vi "Transmit Module Command.vi"(8 "error in":errorcluster, 11 "SL_SC in":refnum<class "SL_SC.lvclass">) -> (0 "error out":errorcluster, 3 "SL_SC out":refnum<class "SL_SC.lvclass">)   [LabVIEW 2019, in "SL_SC.lvlib" / "SL_SC.lvclass"]
uses:
  Library/SL_SC.lvclass
  C:/Users/Public/Documents/Development/builds/Instruments/DIG_IO.lvlibp/Library/DIG_IO.lvclass
  Library/SL_SC.lvclass/SL_SC.ctl
  builds/Instruments/DIG_IO.lvlibp/Accessors/Read Digital.vi
  <vilib>/SLSC/Set Device Property (U32).vi
  <vilib>/SLSC/Commit Properties for Devices.vi
  <vilib>/SLSC/SLSC.lvlib
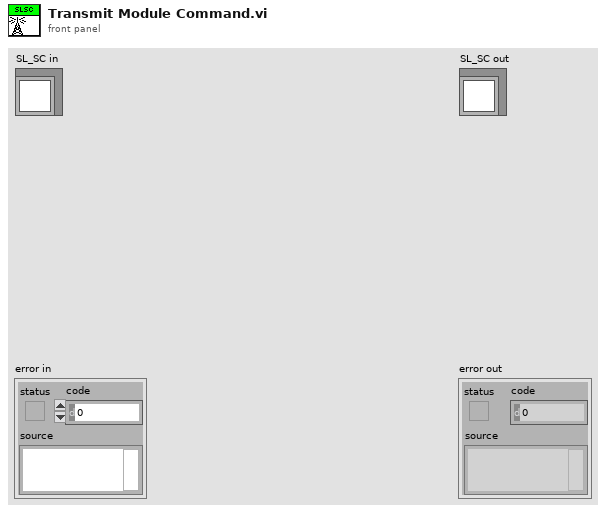
[diagram p1: front panel]
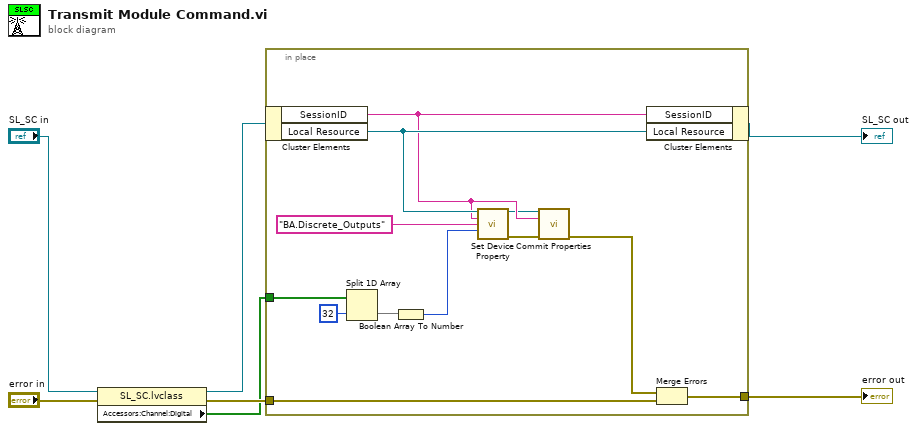
[diagram p0: block diagram]
diagram:
  n1 = property class="SL_SC.lvclass"(reference="SL_SC in", error in="error in") -> (reference out=w2:refnum<class "SL_SC.lvclass">, error out=w4:errorcluster, "Accessors:Channel:Digital"=w1:bool[])
  n2 = in-place {
    in-place-border: w4 -> [w16]
    in-place-border: [w15] -> w5
    in-place-border: w1 -> [w9]
    n3 = in-place-cluster #1(w2) -> ("SessionID"=w18:string, "Local Resource"=w19:refnum<k21>)
    n4 = Split 1D Array(array=w9, index=32) -> (second subarray=w11:bool[])  [unwired: 1 out]
    n5 = Boolean Array To Number(Boolean array=w11) -> (number=w8:u32)
    n6 = call-poly <vilib>:"Set Device Property.vi"("session in"=w19, "devices"=w18, "property"="BA.Discrete_Outputs", "property value"=w8) -> ("session out"=w13:refnum<k21>, "error out"=w12:errorcluster)  [unwired: 10 in]
    n7 = call-poly <vilib>:"Commit Properties.vi"("session in"=w13, "devices"=w18, "error in (no error)"=w12) -> ("error out"=w17:errorcluster)  [unwired: 11 in, 1 out]
    n8 = in-place-cluster #1("SessionID"=w18, "Local Resource"=w19) -> (→"SL_SC out":refnum<class "SL_SC.lvclass">)
    n9 = Merge Errors(w17, w16) -> (w15:errorcluster)
  }
  "error out" <- w5
